vi "launch Panel Manager.vi"   [LabVIEW 2015, in "Panel Manager Controller.lvclass"]
uses:
  Panel Manager Controller.lvclass
  <vilib>/ActorFramework/Actor/Actor.lvclass
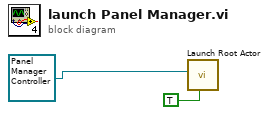
[diagram p0: block diagram]
diagram:
  n1 = call <vilib>:"Launch Root Actor.vi"("Open Actor Core front panel? (F)"=TRUE, "Actor"=refnum<class "Panel Manager Controller.lvclass"> refnum ("Panel Manager Controller.lvclass")) -> ()  [unwired: 8 in, 2 out]
